vi "Calc Heights.vi"(11 "State In":T1) -> (3 "State":T1)   [LabVIEW 2020, in "FlexBlock.xnode"]
uses:
  FlexBlock.xnode
  State.ctl
  FlexBlocks/Type Descriptor.ctl
  FlexBlocks/Terminal Direction.ctl
  FlexBlocks/Value Mode.ctl
  FlexBlocks/Terminal State.ctl
  FlexBlocks/Special Terminal.ctl
  FlexBlocks/Errors.ctl
  <vilib>/picture/picture.llb/imagedata.ctl
  FlexBlocks/Calculated Sizes.ctl
  FlexBlocks/FlexBlocks.lvlib
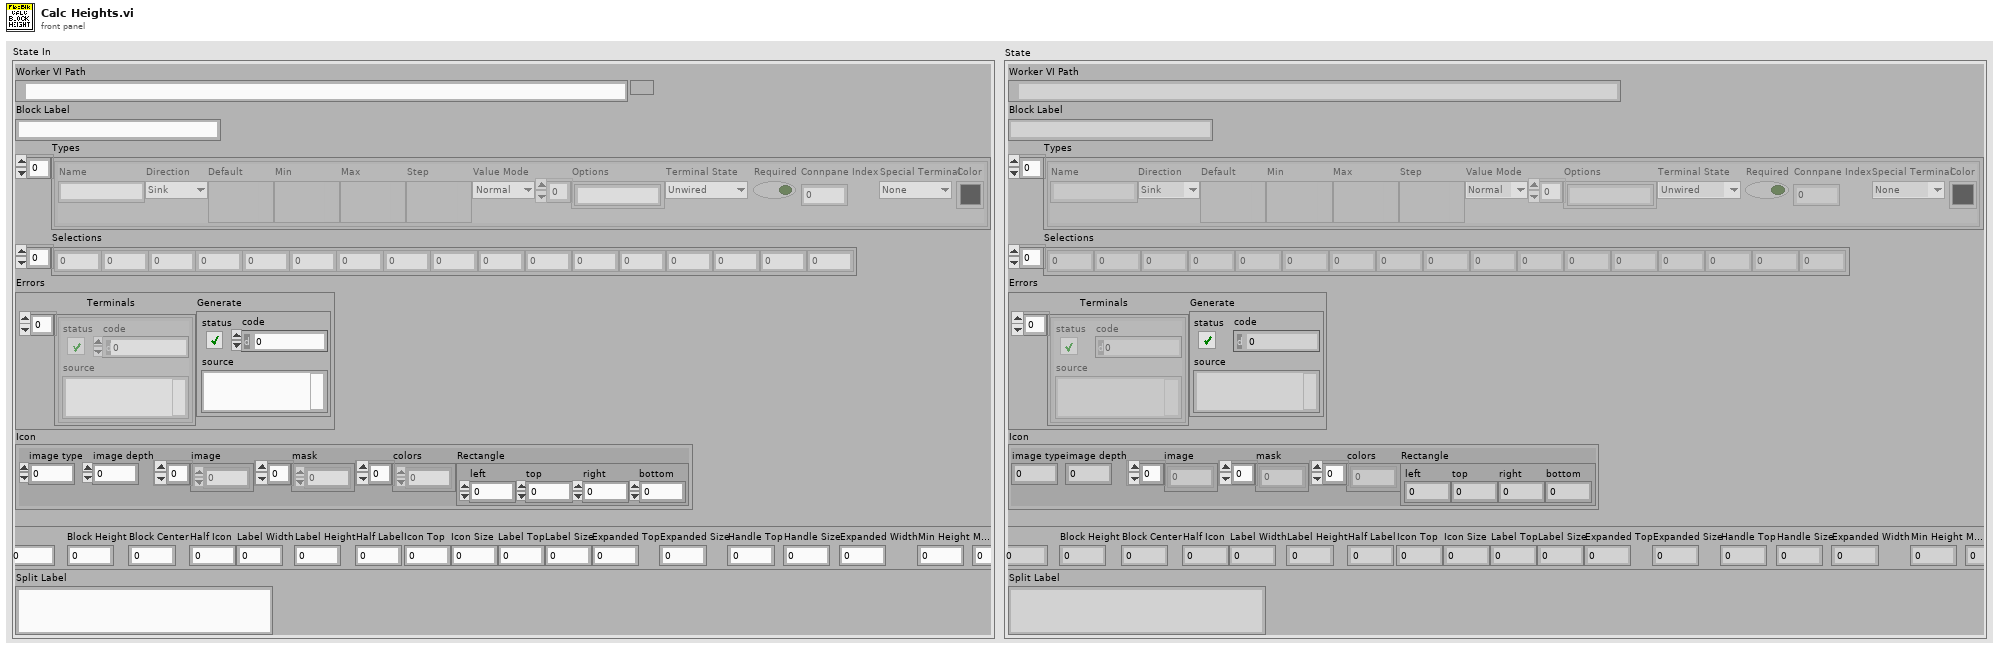
[diagram p1: front panel]
types:
  T1 = typedef "FlexBlock.xnode/State.ctl" = cluster{"Worker VI Path":path, "Block Label":string, "Types":T2[], "Selections":i32[], "Errors":T7, "Icon":T8, "Calcd Sizes":T9, "Split Label":string}
  T2 = typedef "FlexBlocks.lvlib/Type Descriptor.ctl" = cluster{"Name":string, "Direction":T3, "Default":variant, "Min":variant, "Max":variant, "Step":variant, "Value Mode":T4, "Options":string[], "Terminal State":T5, "Required":bool, "Connpane Index":i32, "Special Terminal":T6, "Color":u32}
  T3 = typedef "FlexBlocks.lvlib/Terminal Direction.ctl" = enum16{"Sink", "Source"}
  T4 = typedef "FlexBlocks.lvlib/Value Mode.ctl" = enum16{"Normal", "Range", "Select"}
  T5 = typedef "FlexBlocks.lvlib/Terminal State.ctl" = enum16{"Unwired", "BadType", "BadRef", "Channel", "Value", "Control Ref"}
  T6 = typedef "FlexBlocks.lvlib/Special Terminal.ctl" = enum16{"None", "Action", "Init", "Tag", "State in", "State out", "Error"}
  T7 = typedef "FlexBlocks.lvlib/Errors.ctl" = cluster{"Terminals":errorcluster[], "Generate":errorcluster}
  T8 = typedef "imagedata.ctl" = cluster{"image type":i32, "image depth":i32, "image":u8[], "mask":u8[], "colors":u32[], "Rectangle":cluster{"left":i16, "top":i16, "right":i16, "bottom":i16}}
  T9 = typedef "FlexBlocks.lvlib/Calculated Sizes.ctl" = cluster{"Text Width":i32, "Text Height":i32, "Half Text":i32, "Block Width":i32, "Block Height":i32, "Block Center":i32, "Half Icon":i32, "Label Width":i32, "Label Height":i32, "Half Label":i32, "Icon Top":i32, "Icon Size":i32, "Label Top":i32, "Label Size":i32, "Expanded Top":i32, "Expanded Size":i32, "Handle Top":i32, "Handle Size":i32, "Expanded Width":i32, "Min Height":i32, "Max Height":i32}
  T10 = typedef "FlexBlocks.lvlib/Size Constants.ctl" = cluster{"Icon":i32, "Value Width":i32, "BG Rounding":i32, "Term Width":i32, "Term Height":i32, "Text Offset":i32, "Value Padding":i32, "Select Padding":i32, "Min Block Width":i32, "Vertical Margin":i32, "Size Handle Height":i32}
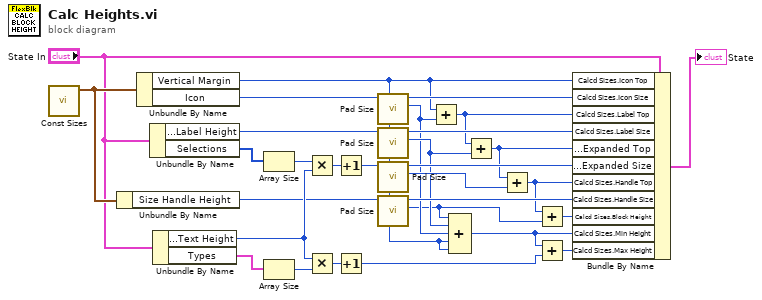
[diagram p0: block diagram]
diagram:
  n1 = call "Const Sizes.vi"() -> ("Sizes"=w25:T10)  [unwired: 11 in]
  n2 = Unbundle By Name(w25) -> ("Size Handle Height"=w12:i32)
  n3 = Unbundle By Name(w25) -> ("Vertical Margin"=w1:i32, "Icon"=w29:i32)
  n4 = Unbundle By Name("State In") -> ("Calcd Sizes.Label Height"=w26:i32, "Selections"=w23:i32[])
  n5 = Unbundle By Name("State In") -> ("Calcd Sizes.Text Height"=w14:i32, "Types"=w16:T2[])
  n6 = Array Size(array=w23) -> (size(s)=w21:i32)
  n7 = Array Size(array=w16) -> (size(s)=w15:i32)
  n8 = Multiply(x=w21, y=w14) -> (x*y=w19:i32)
  n9 = Multiply(x=w14, y=w15) -> (x*y=w4:i32)
  n10 = Increment(x=w19) -> (x+1=w5:i32)
  n11 = Increment(x=w4) -> (x+1=w3:i32)
  n12 = call "Pad Size.vi"("Padding (0)"=w1, "Value"=w29) -> ("Padded or Zero"=w8:i32, "Value or Zero"=w28:i32)  [unwired: 8 in]
  n13 = call "Pad Size.vi"("Padding (0)"=w1, "Value"=w26) -> ("Padded or Zero"=w9:i32, "Value or Zero"=w27:i32)  [unwired: 8 in]
  n14 = call "Pad Size.vi"("Padding (0)"=w1, "Value"=w5) -> ("Padded or Zero"=w17:i32, "Value or Zero"=w20:i32)  [unwired: 8 in]
  n15 = call "Pad Size.vi"("Padding (0)"=w1, "Value"=w12) -> ("Padded or Zero"=w2:i32, "Value or Zero"=w13:i32)  [unwired: 8 in]
  n16 = Add(x=w1, y=w8) -> (x+y=w24:i32)
  n17 = Compound Arithmetic op=ADD(w2, w9, w8, w1, w1) -> (w6:i32)
  n18 = Add(x=w24, y=w9) -> (x+y=w18:i32)
  n19 = Add(x=w18, y=w17) -> (x+y=w10:i32)
  n20 = Add(x=w10, y=w2) -> (x+y=w11:i32)
  n21 = Add(x=w6, y=w3) -> (x+y=w7:i32)
  n22 = Bundle By Name(cluster="State In", "Calcd Sizes.Icon Top"=w1, "Calcd Sizes.Icon Size"=w28, "Calcd Sizes.Label Top"=w24, "Calcd Sizes.Label Size"=w27, "Calcd Sizes.Expanded Top"=w18, "Calcd Sizes.Expanded Size"=w20, "Calcd Sizes.Handle Top"=w10, "Calcd Sizes.Handle Size"=w13, "Calcd Sizes.Block Height"=w11, "Calcd Sizes.Min Height"=w6, "Calcd Sizes.Max Height"=w7) -> (→"State":T1)
